vi "FPGA_DIOWriteFilterSelect.vi"(8 "error in (no error)":errorcluster, 9 "PWMFilterSelect":u8, 10 "channel index":u8, 11 "DIODeviceRef":T1) -> (0 "error out":errorcluster, 3 "DIODeviceRef":T1)   [LabVIEW 2017]
uses:
  <vilib>/Rock Robotics/SystemInterfaces/DIO/FPGA_DIODevRef.ctl
  <vilib>/Rock Robotics/SystemInterfaces/System/FPGA_SystemFPGA Ref Global.vi
  <vilib>/Utility/error.llb/Error Cluster From Error Code.vi
  <vilib>/rvi/errors/niLvFpgaAdjustHostInterfaceError.vi
  <vilib>/rvi/interface/nirviReadWriteControl/nirviReadWriteControl.xnode
  <vilib>/Rock Robotics/SystemInterfaces/System/FPGA_SystemFRC FPGA Ref.ctl
  NiFpgaLv.dll
  <vilib>/rvi/interface/Simulation/niFpgaSimulationCallBeginRW.vi
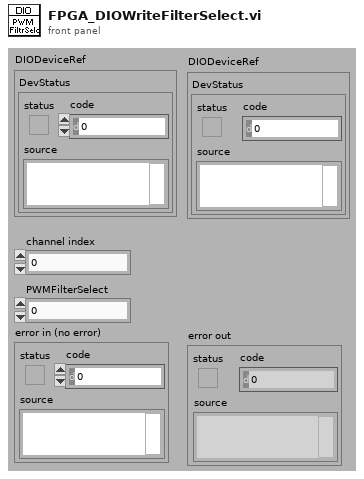
[diagram p1: front panel]
types:
  T1 = typedef "FPGA_DIODevRef.ctl" = cluster{"DevStatus":errorcluster}
  T2 = typedef "FPGA_SystemFRC FPGA Ref.ctl" = refnum<k20>
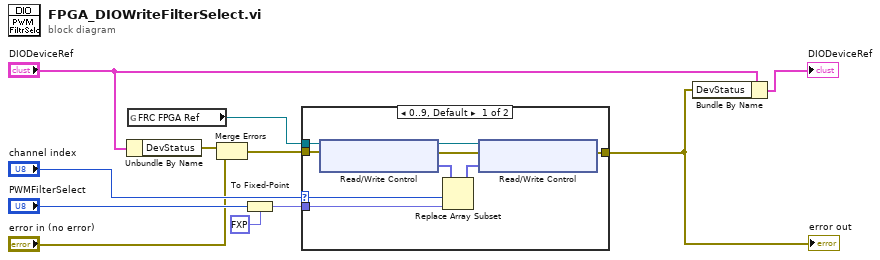
[diagram p0: block diagram]
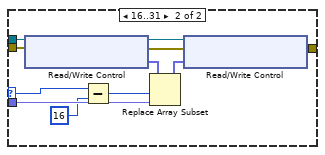
[diagram p2: hidden frame]
diagram:
  n1 = Unbundle By Name("DIODeviceRef") -> ("DevStatus"=w3:errorcluster)
  n2 = global read "FPGA_SystemFPGA Ref Global.vi" "FRC FPGA Ref"() -> (w4:T2)
  n3 = Merge Errors(w3, "error in (no error)") -> (w2:errorcluster)
  n4 = To Fixed-Point(fixed-point type=fxp<+,2,2> 0.0 ("new element/subarray"), number="PWMFilterSelect") -> (fixed-point=w6:fxp<+,2,2>)
  n5 = case shown="0..9, Default" "channel index" {
    selector: "channel index" -> [w12 w22]
    tunnel: [w19 w30] -> w8
    tunnel: w6 -> [w17 w28]
    tunnel: w2 -> [w15 w26]
    tunnel: w4 -> [w14 w25]
    frame 0..9, Default {
      n6 = xnode "Read/Write Control"("FPGA VI Reference In"=w14, "error in"=w15) -> ("FPGA VI Reference Out"=w20:T2, "error out"=w16:errorcluster, "DIO.FilterSelectHdr"=w13:fxp<+,2,2>[])
      n7 = Replace Array Subset(array=w13, new element=w17, index=w12) -> (w18:fxp<+,2,2>[])
      n8 = xnode "Read/Write Control"("FPGA VI Reference In"=w20, "error in"=w16, "DIO.FilterSelectHdr"=w18) -> ("error out"=w19:errorcluster)  [unwired: 1 out]
    }
    frame 16..31 {
      n9 = xnode "Read/Write Control"("FPGA VI Reference In"=w25, "error in"=w26) -> ("FPGA VI Reference Out"=w31:T2, "error out"=w27:errorcluster, "DIO.FilterSelectMXP"=w24:fxp<+,2,2>[])
      n10 = Subtract(x=w22, y=u8 16) -> (x-y=w21:u8)
      n11 = Replace Array Subset(array=w24, new element=w28, index=w21) -> (w29:fxp<+,2,2>[])
      n12 = xnode "Read/Write Control"("FPGA VI Reference In"=w31, "error in"=w27, "DIO.FilterSelectMXP"=w29) -> ("error out"=w30:errorcluster)  [unwired: 1 out]
    }
  }
  "error out" <- w8
  n13 = Bundle By Name(cluster="DIODeviceRef", "DevStatus"=w8) -> (→"DIODeviceRef":T1)
